vi "publisher tests Reader.vi"() -> ()   [LabVIEW 2018]
uses:
  publisher action.ctl
panel:
  in  "Boolean":bool
  out "number":dbl
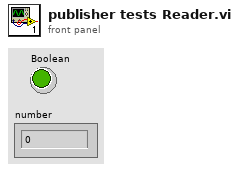
[diagram p1: front panel]
types:
  T1 = typedef "publisher action.ctl" = enum16{"set", "get", "init", "--send request", "--wait", "--respond", "init writer", "init reader"}
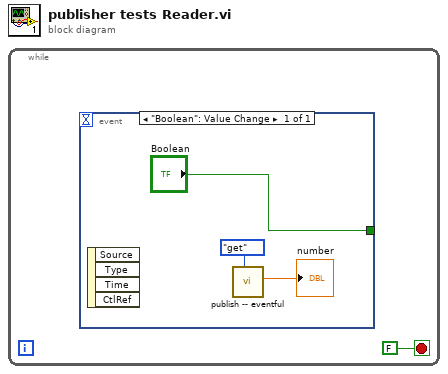
[diagram p0: block diagram]
diagram:
  n1 = while {
    stop <- FALSE stop-if-true
    n2 = event shown="[0] \"Boolean\": Value Change" {
      selector: _ -> [_]
      dyn-events: _ -> [_]
      timeout: _ -> [_]
      tunnel: ["Boolean"] -> _
      event "Boolean": Value Change {
        n3 = event-data() -> ()  [unwired: 1 in, 4 out]
        n4 = call "publish -- eventful.vi"("publisher action"=publisher_action."get") -> ("stepper pos OUT"=→"number":dbl)  [unwired: 8 in, 2 out]
      }
    }
  }
